vi "Write acquisition type (Normal).vi"(8 "error in (no error)":errorcluster, 10 "acquisition type (Normal)":i32(ring) items=["Normal", "Peak Detect", "High Resolution", "Envelope", "Average"], 11 "Configure Acquisition Type Msg in":refnum<class "Configure Acquisition Type Msg.lvclass">) -> (0 "error out":errorcluster, 3 "Configure Acquisition Type Msg out":refnum<class "Configure Acquisition Type Msg.lvclass">)   [LabVIEW 2014, in "CS++Scope.lvlib" / "Configure Acquisition Type Msg.lvclass"]
uses:
  Configure Acquisition Type Msg.lvclass
  Configure Acquisition Type Msg.lvclass/Configure Acquisition Type Msg.ctl
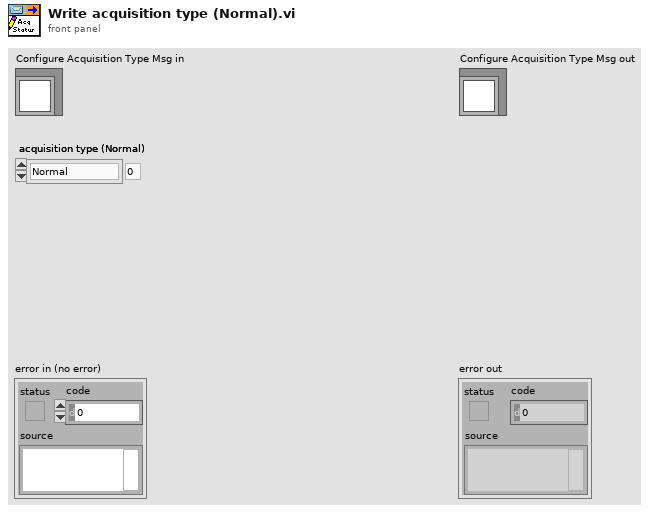
[diagram p1: front panel]
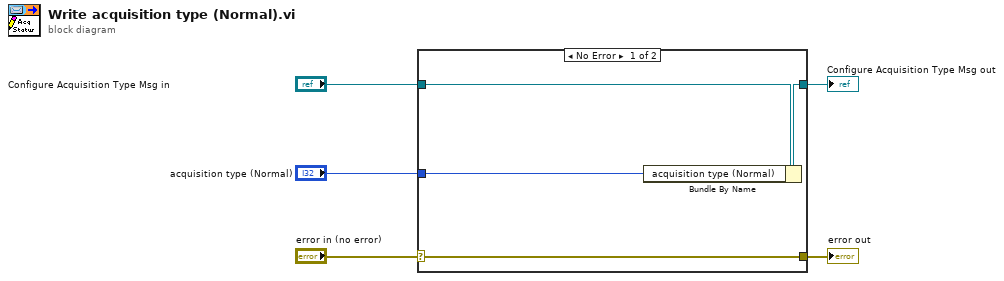
[diagram p0: block diagram]
diagram:
  n1 = case shown="No Error" "error in (no error)" {
    selector: "error in (no error)" -> [w9 w10]
    tunnel: [w9 w10] -> w4
    tunnel: [w7 w11] -> w2
    tunnel: "Configure Acquisition Type Msg in" -> [w8 w11]
    tunnel: "acquisition type (Normal)" -> [w6 _]
    frame No Error {
      n2 = Bundle By Name(cluster=w8, "acquisition type (Normal)"=w6) -> (w7:refnum<class "Configure Acquisition Type Msg.lvclass">)
    }
    frame Error {
    }
  }
  "error out" <- w4
  "Configure Acquisition Type Msg out" <- w2
